vi "create file object.vi"(8 "error in":errorcluster, 11 "file path":path) -> (0 "error out":errorcluster, 3 "reference out":refnum<class "File.lvclass">)   [LabVIEW 2023, in "File Classes.lvlib"]
uses:
  File Classes.lvlib
  File/File.lvclass
  Picture File/Picture File.lvclass
  Video File/Video File.lvclass
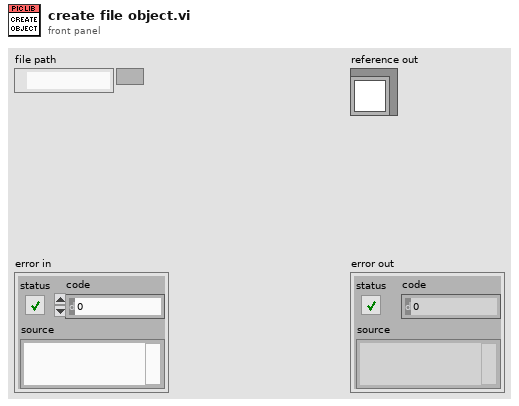
[diagram p1: front panel]
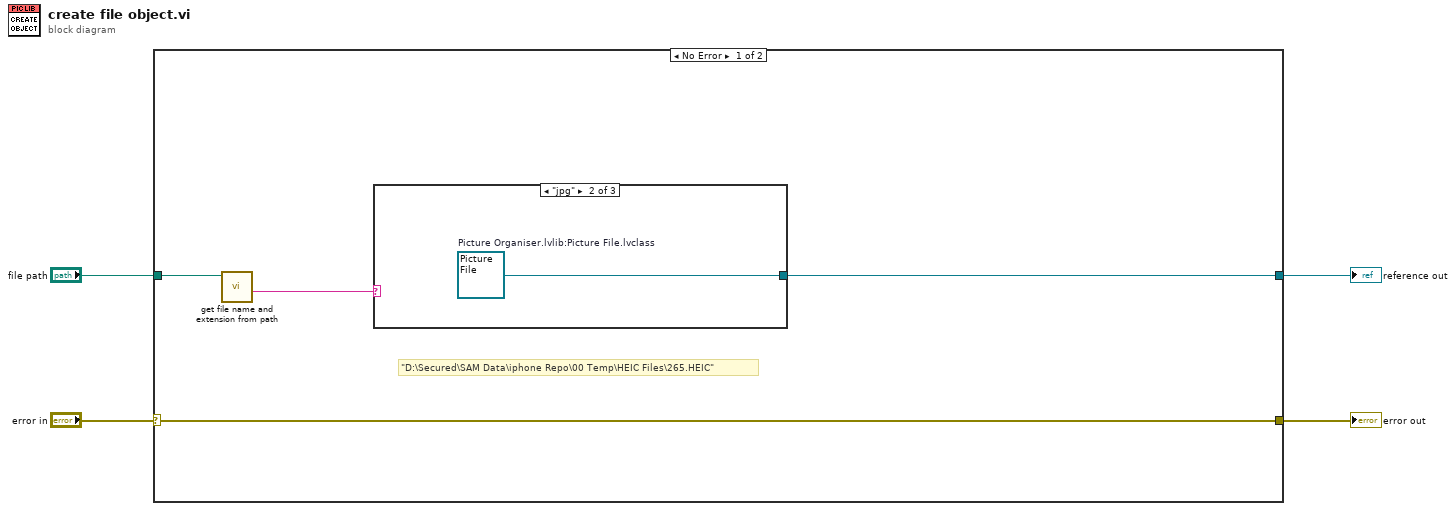
[diagram p0: block diagram]
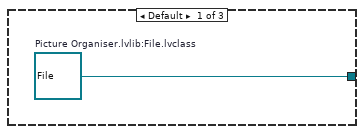
[diagram p2: hidden frame]
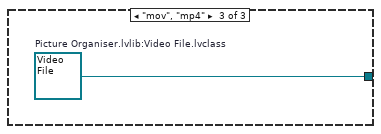
[diagram p3: hidden frame]
diagram:
  n1 = case shown="No Error" "error in" {
    selector: "error in" -> [w5 w12]
    tunnel: "file path" -> [w8 _]
    tunnel: [w6 _] -> w3
    tunnel: [w5 w12] -> w1
    frame No Error {
      # "\"D:\\Secured\\SAM Data\\iphone Repo\\00 Temp\\HEIC Files\\265.HEIC\""
      n2 = call "get file name and extension from path.vi"("fiel path"=w8) -> ("file extension"=w7:string)  [unwired: 8 in, 2 out]
      n3 = case shown="\"jpg\"" w7 {
        tunnel: [w9 w10 w11] -> w6
        frame Default {
          w9 = refnum<class "File.lvclass"> refnum  # Picture Organiser.lvlib:File.lvclass
        }
        frame "jpg" {
          w10 = refnum<class "Picture File.lvclass"> refnum  # Picture Organiser.lvlib:Picture File.lvclass
        }
        frame "mov", "mp4" {
          w11 = refnum<class "Video File.lvclass"> refnum  # Picture Organiser.lvlib:Video File.lvclass
        }
      }
    }
    frame Error {
    }
  }
  "reference out" <- w3
  "error out" <- w1
